vi "Keyence.Example.Read.vi"() -> ()   [LabVIEW 2015]
uses:
  LowLevel/Keyence.CodeDetails.ctl
panel:
  in  "Bank":u8=1
  out "model":string
  out "Code":T1
  out "error out":errorcluster
  in  "IP":string="192.168.100.5"
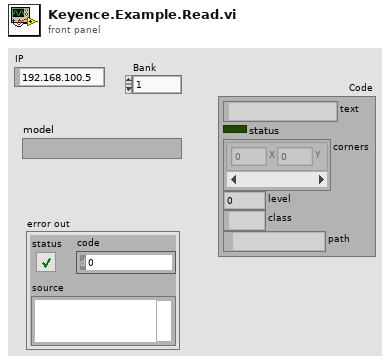
[diagram p1: front panel]
types:
  T1 = typedef "Keyence.CodeDetails.ctl" = cluster{"text":string, "status":bool, "corners":cluster{"X":i32, "Y":i32}[], "level":u8, "class":string, "path":path}
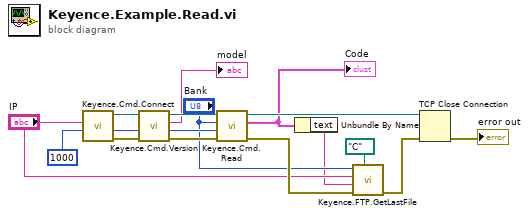
[diagram p0: block diagram]
diagram:
  w9 = 1000 ("Timeout [ms] (1000)")
  n1 = call "Keyence.Cmd.Connect.vi"("Timeout [ms] (1000)"=w9, "IP"="IP") -> ("error out"=w15:errorcluster, "connection ID out"=w14:refnum<k5>)  [unwired: 8 in]
  n2 = call "Keyence.Cmd.Version.vi"("error in (no error)"=w15, "Timeout [ms] (1000)"=w9, "connection ID"=w14) -> ("error out"=w10:errorcluster, "model"=→"model":string, "connection ID out"=w13:refnum<k5>)  [unwired: 4 in, 2 out]
  n3 = call "Keyence.Cmd.Read.vi"("error in (no error)"=w10, "Timeout [ms] (1000)"=w9, "Bank"="Bank", "connection ID"=w13) -> ("error out"=w7:errorcluster, "Code"=w3:T1, "connection ID out"=w11:refnum<k5>)  [unwired: 4 in, 1 out]
  "Code" <- w3
  n4 = Unbundle By Name(w3) -> ("text"=w2:string)
  n5 = call "Keyence.FTP.GetLastFile.vi"("LogPath"=path "C:/", "error in (no error)"=w7, "Name (temp)"=w2, "host"="IP", "Bank (0)"="Bank") -> ("error out"=w6:errorcluster)  [unwired: 4 in, 2 out]
  n6 = TCP Close Connection(connection ID=w11, error in (no error)=w6) -> (error out=→"error out":errorcluster)  [unwired: 1 in, 1 out]
